vi "Split Registers by Direction.vi"(8 "error in":errorcluster, 11 "vi info":T1 {"RegisterMap"."Address" format="%.0x"}) -> (0 "error out":errorcluster, 2 "Controls":T8[](array[typedef]) {"Data Type" format="%.0x"}, 3 "Indicator":T8[](array[typedef]) {"Data Type" format="%.0x"})   [LabVIEW 2019, in "FPGA Addon System Explorer.lvlib"]
uses:
  FPGA Addon System Explorer.lvlib
  Shared/Register Information.ctl
  Shared/Data Type.ctl
  <vilib>/rvi/Bitfile/niFpgaBitfileStructure_VI.ctl
  <vilib>/rvi/Bitfile/nirviControlStructure.ctl
  <vilib>/rvi/Bitfile/nirviTypdefDescription.ctl
  <vilib>/rvi/Bitfile/nirviMechanicalAction.ctl
  <vilib>/rvi/Bitfile/nirviSubControlStructure.ctl
  <vilib>/rvi/Bitfile/nirviClusterElementControl.ctl
  <vilib>/picture/picture.llb/imagedata.ctl
  SubModules/FPGA Addon Speciality IO/Source/Types/PWM.Measure.Analog.Measurement.ctl
  SubModules/FPGA Addon Speciality IO/Source/Types/PWM.Measure.Digital.Measurement.ctl
  SubModules/FPGA Addon Speciality IO/Source/Types/Static.Measure.Digital.Measurement.ctl
  SubModules/FPGA Addon Speciality IO/Source/Types/QuadratureEncoder.Measure.Digital.Measurement.ctl
  SubModules/FPGA Addon Speciality IO/Source/Types/PWM.Generate.Digital.Settings.ctl
  SubModules/FPGA Addon Speciality IO/Source/Types/PWM.Measure.Analog.Settings.ctl
  SubModules/FPGA Addon Speciality IO/Source/Types/PWM.Measure.Digital.Settings.ctl
  SubModules/FPGA Addon Speciality IO/Source/Types/Sine.Generate.Settings.ctl
  SubModules/FPGA Addon Speciality IO/Source/Types/Static.Generate.Digital.Settings.ctl
  SubModules/FPGA Addon Speciality IO/Source/Types/Static.Measure.Digital.Settings.ctl
  SubModules/FPGA Addon Speciality IO/Source/Types/WSS.Generate.Digital.Settings.ctl
  SubModules/FPGA Addon Speciality IO/Source/Types/QuadratureEncoder.Measure.Digital.Settings.ctl
  Shared/FPGA Addon Shared.lvlib
  SubModules/FPGA Addon Speciality IO/Source/Speciality FPGA IO.lvlib
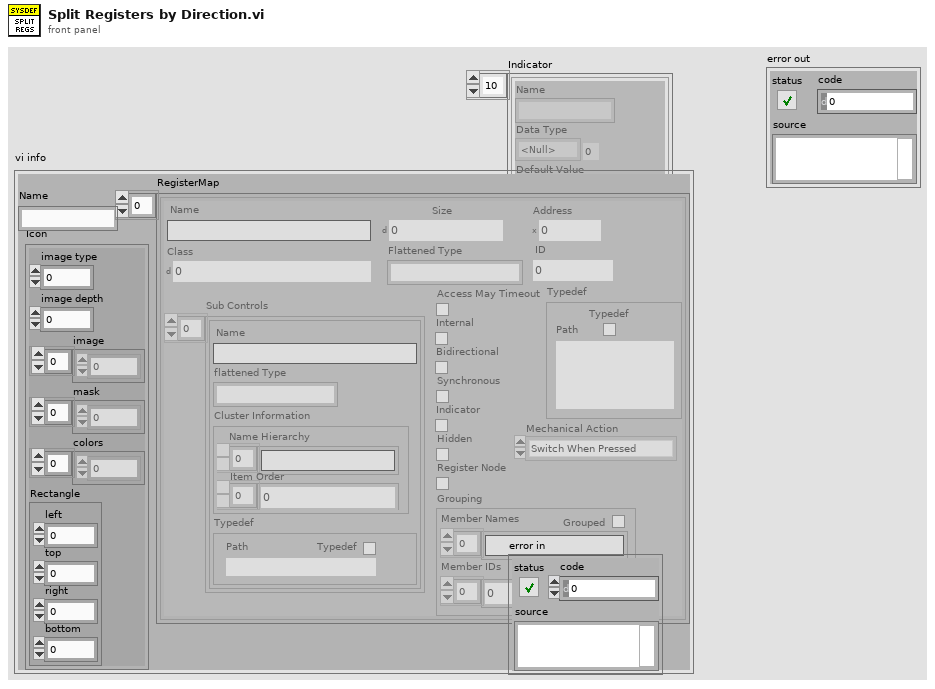
[diagram p1: front panel]
types:
  T1 = typedef "niFpgaBitfileStructure_VI.ctl" = cluster{"Name":string, "RegisterMap":T2[], "Icon":T7}
  T2 = typedef "nirviControlStructure.ctl" = cluster{"Name":string, "Hidden":bool, "Indicator":bool, "Flattened Type":string, "Grouping":cluster{"Grouped":bool, "Member Names":string[], "Member IDs":u32[]}, "Address":u32, "Size":u32, "Class":u32, "Internal":bool, "Typedef":T3, "ID":u32, "Bidirectional":bool, "Synchronous":bool, "Mechanical Action":T4, "Sub Controls":T5[], "Access May Timeout":bool, "Register Node":bool}
  T3 = typedef "nirviTypdefDescription.ctl" = cluster{"Typedef":bool, "Path":path}
  T4 = typedef "nirviMechanicalAction.ctl" = enum8{"Switch When Pressed", "Switch When Released", "Switch Until Released", "Latch When Pressed", "Latch When Released", "Latch Until Released"}
  T5 = typedef "nirviSubControlStructure.ctl" = cluster{"Name":string, "flattened Type":string, "Cluster Information":T6, "Typedef":T3}
  T6 = typedef "nirviClusterElementControl.ctl" = cluster{"Name Hierarchy":string[], "Item Order":u32[]}
  T7 = typedef "imagedata.ctl" = cluster{"image type":i32, "image depth":i32, "image":u8[], "mask":u8[], "colors":u32[], "Rectangle":cluster{"left":i16, "top":i16, "right":i16, "bottom":i16}}
  T8 = typedef "FPGA Addon Shared.lvlib/Register Information.ctl" = cluster{"Name":string, "Data Type":T9, "Default Value":variant}
  T9 = typedef "FPGA Addon Shared.lvlib/Data Type.ctl" = enum8{"<Null>", "I8", "I16", "I32", "I64", "U8", "U16", "U32", "U64", "SGL", "Boolean", "Analog PWM In Settings", "Analog PWM In", "Digital PWM In Settings", "Digital PWM In", "Digital PWM Out", "Sine Out", "FXP+/-24.5", "FXP+/-16.5", "FXP+/-32.8", "FXP+/-64.32", "FXP+/-16.7", "FXP+/-20.5", "FXP+/-27.5", "FXP+/-32.16", "FXP +16.3", "FXP +18.3", "Digital Static In", "Digital Static Out", "Digital Static In Settings", "Digital WSS Out", "Quad Encoder Settings", "Quad Encoder In"}
  T10 = typedef "Speciality FPGA IO.lvlib/QuadratureEncoder.Measure.Digital.Measurement.ctl" = cluster{"POSITION":i32}
  T11 = typedef "Speciality FPGA IO.lvlib/Static.Measure.Digital.Measurement.ctl" = cluster{"STATE":bool}
  T12 = typedef "Speciality FPGA IO.lvlib/PWM.Measure.Digital.Measurement.ctl" = cluster{"ACTIVE TICKS":u32, "INACTIVE TICKS":u32, "ACQ TICKS":u32}
  T13 = typedef "Speciality FPGA IO.lvlib/PWM.Measure.Analog.Measurement.ctl" = cluster{"ACTIVE TICKS":u32, "INACTIVE TICKS":u32, "ACQ TICKS":u32, "ACTIVE VOLTAGE":fxp<+/-,32,8>, "INACTIVE VOLTAGE":fxp<+/-,32,8>}
  T14 = typedef "Speciality FPGA IO.lvlib/QuadratureEncoder.Measure.Digital.Settings.ctl" = cluster{"DIRECTION":u8, "RESET VALUE":i32, "A RESET STATE":bool, "B RESET STATE":bool, "Z RESET STATE":bool}
  T15 = typedef "Speciality FPGA IO.lvlib/WSS.Generate.Digital.Settings.ctl" = cluster{"ACTIVE EDGE":bool, "ACTIVE TICKS":u32, "INACTIVE TICKS":u32, "DATA":u8, "SENSOR TYPE":u8}
  T16 = typedef "Speciality FPGA IO.lvlib/Static.Measure.Digital.Settings.ctl" = cluster{"ACTIVE EDGE":bool}
  T17 = typedef "Speciality FPGA IO.lvlib/Static.Generate.Digital.Settings.ctl" = cluster{"ACTIVE EDGE":bool, "OUTPUT":bool}
  T18 = typedef "Speciality FPGA IO.lvlib/Sine.Generate.Settings.ctl" = cluster{"AMP":fxp<+/-,32,8>, "OFFSET":fxp<+/-,32,8>, "PERIODS/TICKS":fxp<+,32,0>}
  T19 = typedef "Speciality FPGA IO.lvlib/PWM.Measure.Digital.Settings.ctl" = cluster{"ACTIVE EDGE":bool, "TIMEOUT":u32}
  T20 = typedef "Speciality FPGA IO.lvlib/PWM.Measure.Analog.Settings.ctl" = cluster{"ACTIVE EDGE":bool, "TIMEOUT":u32, "THRESHOLD":fxp<+/-,32,8>}
  T21 = typedef "Speciality FPGA IO.lvlib/PWM.Generate.Digital.Settings.ctl" = cluster{"ACTIVE EDGE":bool, "ACTIVE TICKS":u32, "INACTIVE TICKS":u32}
  T22 = typedef "Type Descriptor Enumeration__ogtk.ctl" = enum8{"<Null>", "I8", "I16", "I32", "I64", "U8", "U16", "U32", "U64", "SGL", "DBL", "EXT", "CSG", "CDB", "CXT", "0x0F", "0x10", "0x11", "0x12", "0x13", "0x14", "Enum U8", "Enum U16", "Enum U32", "Enum U64", "SGL PQ", "DBL PQ", "EXT PQ", "CSG PQ", "CDB PQ", "CXT PQ", "0x1F", "0x20", "Boolean", "0x22", "0x23", "0x24", "0x25", "0x26", "0x27", "0x28", "0x29", "0x2A", "0x2B", "0x2C", "0x2D", "0x2E", "0x2F", "String", "0x31", "Path", "Pict", "0x34", "0x35", "0x36", "DAQ", "0x38", "0x39", "0x3A", "0x3B", "0x3C", "0x3D", "0x3E", "0x3F", "Array", "0x41", "0x42", "0x43", "0x44", "0x45", "0x46", "0x47", "0x48", "0x49", "0x4A", "0x4B", "0x4C", "0x4D", "0x4E", "0x4F", "Cluster", "0x51", "0x52", "Variant", "Waveform", "0x55", "0x56", "0x57", "0x58", "0x59", "0x5A", "0x5B", "0x5C", "0x5D", "0x5E", "0x5F", "0x60", "0x61", "0x62", "0x63", "0x64", "0x65", "0x66", "0x67", "0x68", "0x69", "0x6A", "0x6B", "0x6C", "0x6D", "0x6E", "0x6F", "Refnum"}
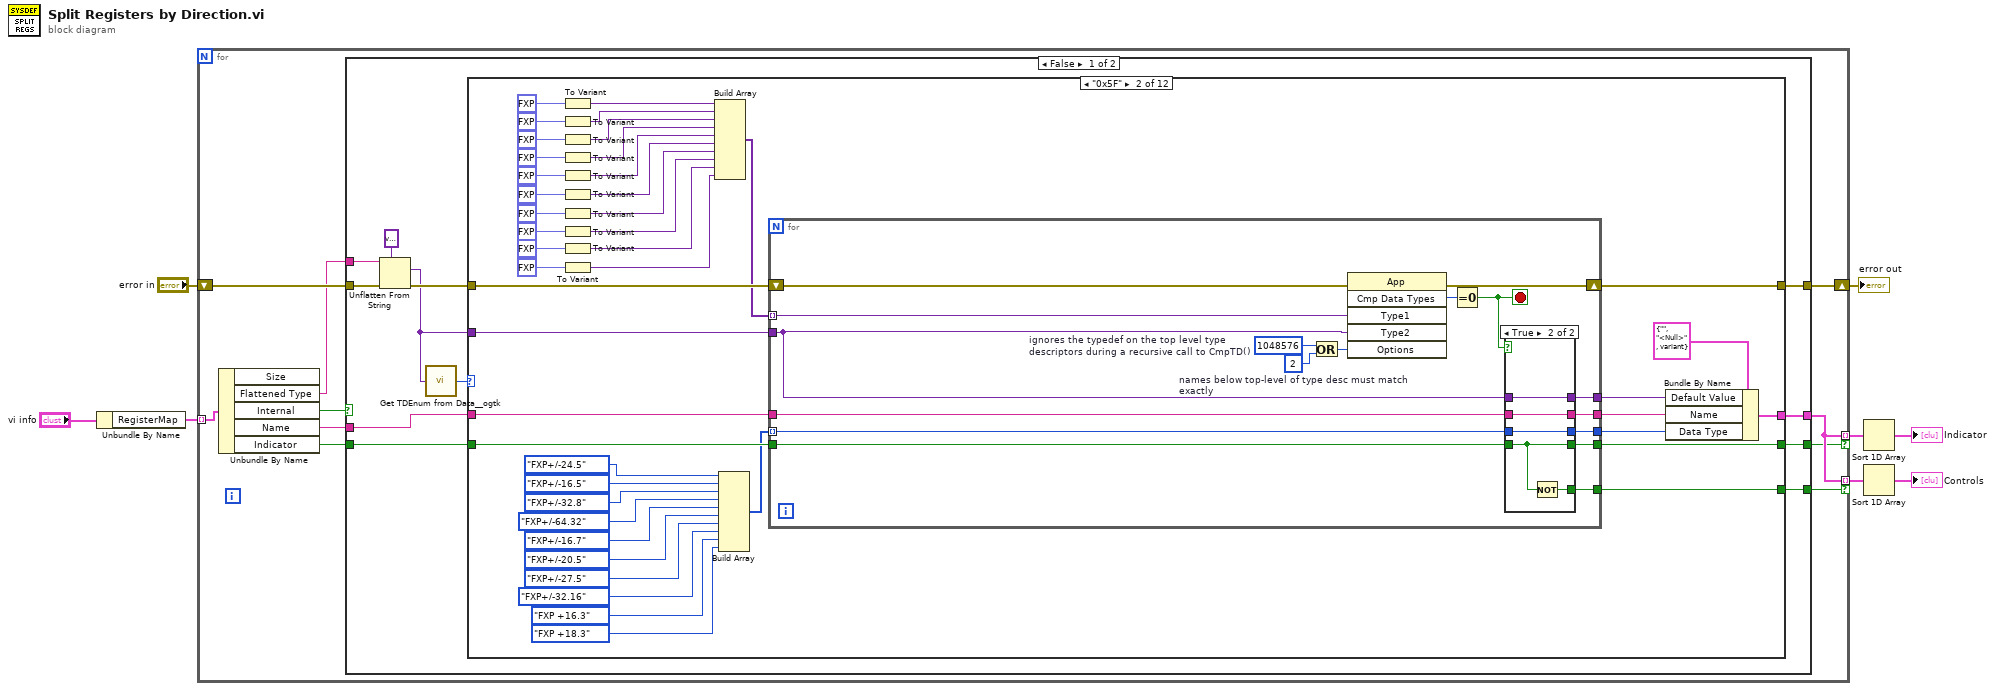
[diagram p0: block diagram]
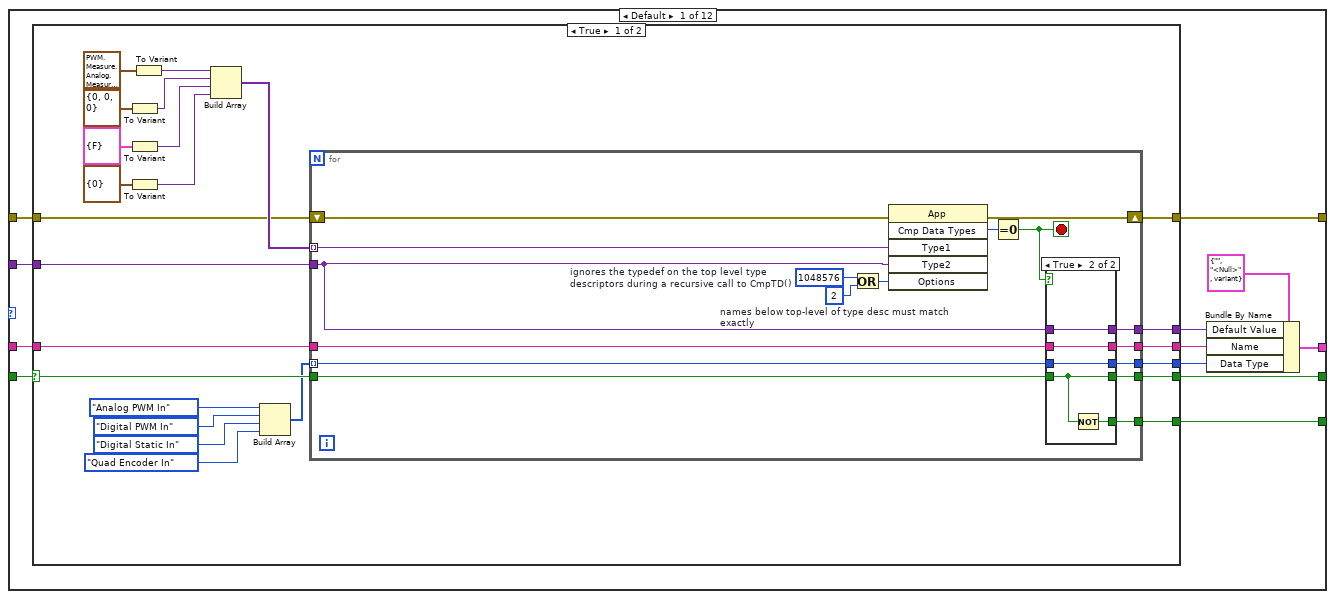
[diagram p2: hidden frame]
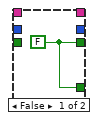
[diagram p3: hidden frame]
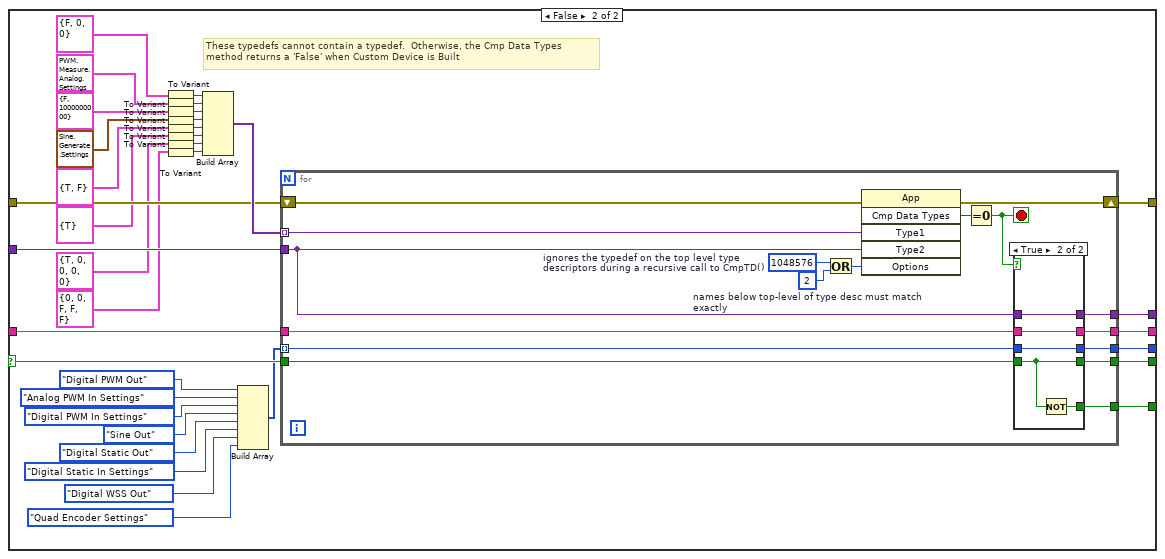
[diagram p4: hidden frame]
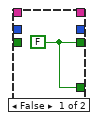
[diagram p5: hidden frame]
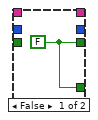
[diagram p6: hidden frame]
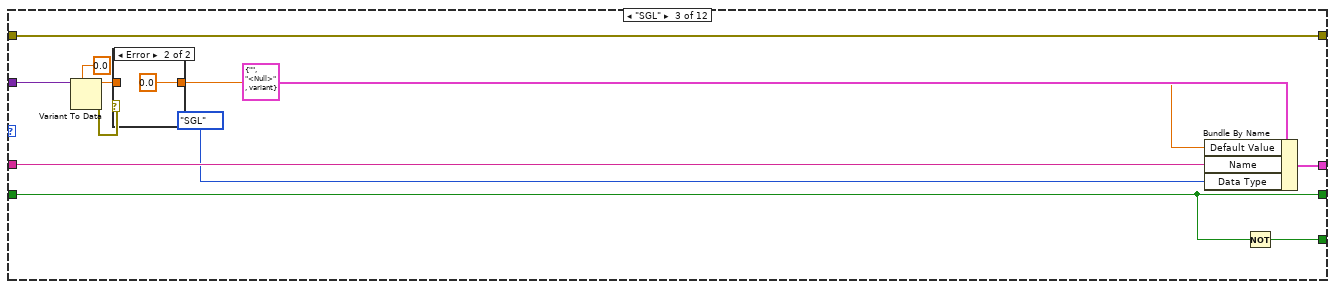
[diagram p7: hidden frame]
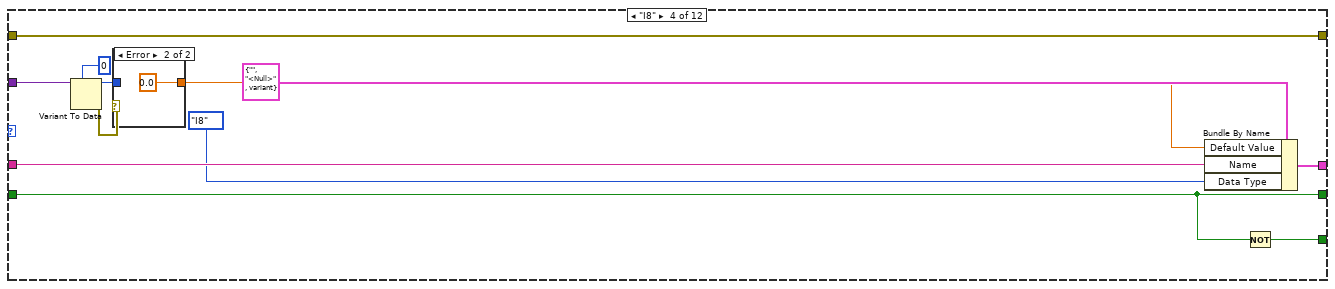
[diagram p9: hidden frame]
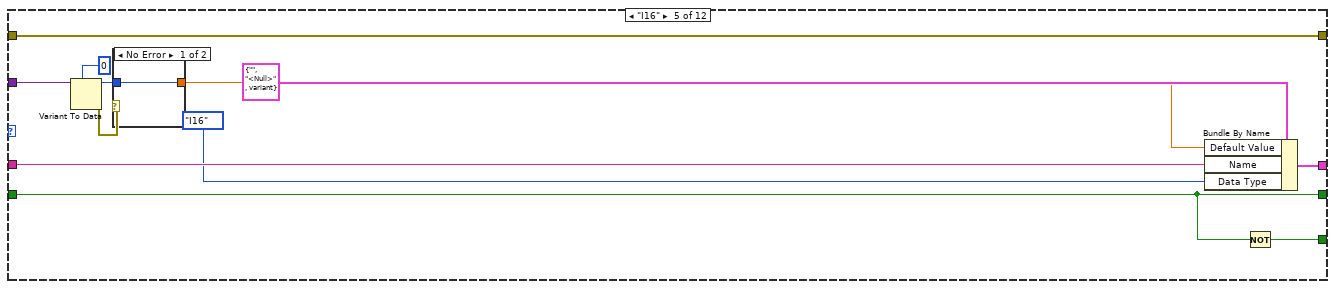
[diagram p11: hidden frame]
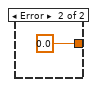
[diagram p12: hidden frame]
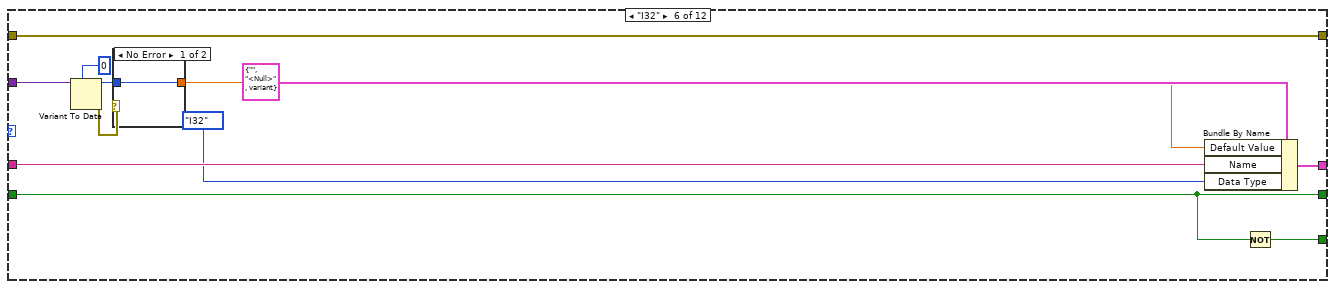
[diagram p13: hidden frame]
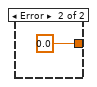
[diagram p14: hidden frame]
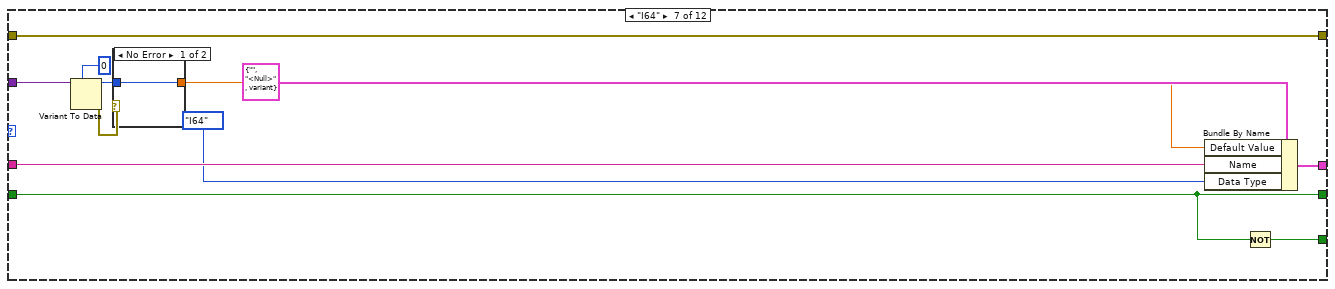
[diagram p15: hidden frame]
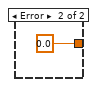
[diagram p16: hidden frame]
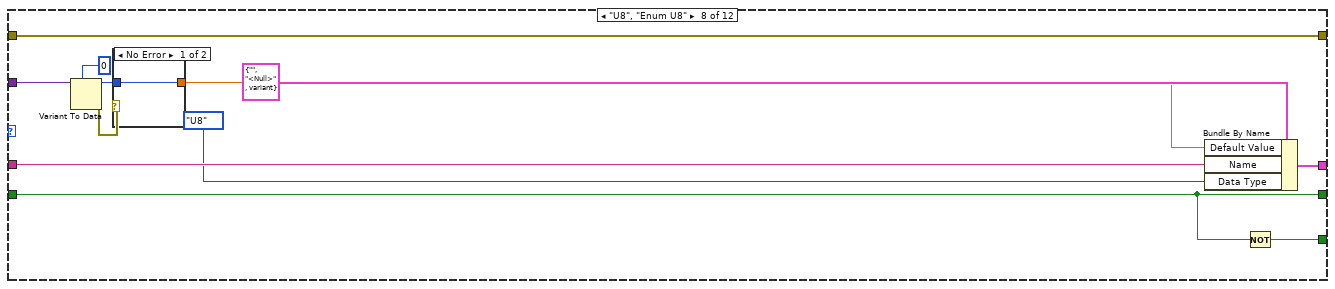
[diagram p17: hidden frame]
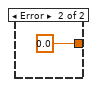
[diagram p18: hidden frame]
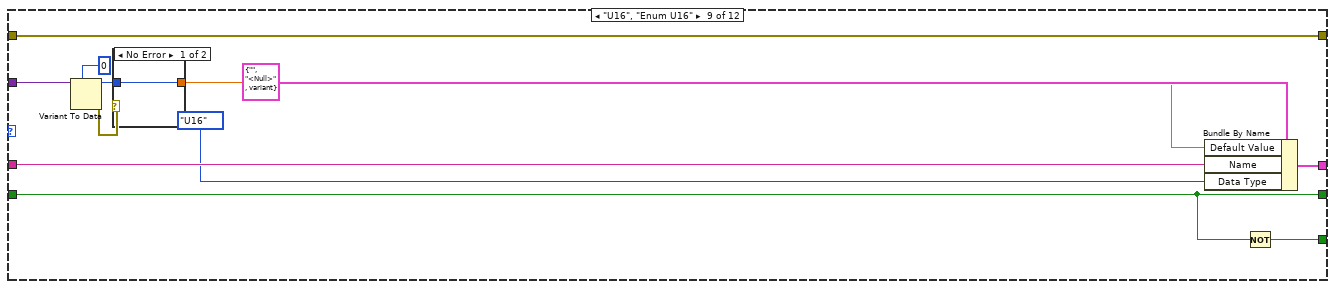
[diagram p19: hidden frame]
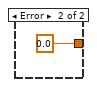
[diagram p20: hidden frame]
diagram:
  n1 = Unbundle By Name("vi info") -> ("RegisterMap"=w6:T2[])
  n2 = for {
    tunnel: w6 -> [w13] mode=indexing
    tunnel: [w18] -> w7 mode=indexing if=w17
    tunnel: [w18] -> w8 mode=indexing if=w16
    shift-right: [w15] -> w2
    shift-left: "error in" -> [w14]
    n3 = Unbundle By Name(w13) -> ("Flattened Type"=w9:string, "Internal"=w10:bool, "Name"=w11:string, "Indicator"=w12:bool)  [unwired: 1 out]
    n4 = case shown="False" w10 {
      tunnel: w11 -> [w29 _]
      tunnel: w12 -> [w28 _]
      tunnel: [w27 _] -> w18
      tunnel: [w26 w358] -> w17
      tunnel: [w25 w358] -> w16
      tunnel: w9 -> [w22 _]
      tunnel: [w24 w357] -> w15
      tunnel: w14 -> [w21 w357]
      frame False {
        n5 = Unflatten From String(type=variant ("Variant"), binary string=w22, error in (no error)=w21) -> (value=w19:variant, error out=w20:errorcluster)  [unwired: 3 out]
        n6 = call <userlib>:"Get TDEnum from Data__ogtk.vi"("Data"=w19) -> ("Type Descriptor Enumeration"=w30:T22)  [unwired: 4 in]
        n7 = case shown="\"0x5F\"" w30 {
          tunnel: [w42 w192 w224 w238 w252 w266 w280 w294 w308 w322 w336 w350] -> w26
          tunnel: w28 -> [w37 w187 w224 w238 w252 w266 w280 w294 w308 w322 w336 w350]
          tunnel: w29 -> [w38 w188 w226 w240 w254 w268 w282 w296 w310 w324 w338 w352]
          tunnel: [w39 w189 w225 w239 w253 w267 w281 w295 w309 w323 w337 w351] -> w27
          tunnel: [w41 w191 w223 w237 w251 w265 w279 w293 w307 w321 w335 w349] -> w25
          tunnel: w19 -> [w36 w186 w222 w236 w250 w264 w278 w292 w306 w320 w334 w348]
          tunnel: [w32 w182 w216 w230 w244 w258 w272 w286 w300 w314 w328 w342] -> w24
          tunnel: w20 -> [w31 w181 w216 w230 w244 w258 w272 w286 w300 w314 w328 w342]
          frame Default {
            n8 = case shown="True" w37 {
              selector: w37 -> [w61 w121]
              tunnel: [w66 w125] -> w42
              tunnel: [w65 w124] -> w41
              tunnel: w38 -> [w64 w123]
              tunnel: w36 -> [w55 w117]
              tunnel: [w54 w116] -> w35
              tunnel: [w53 w115] -> w34
              tunnel: [w52 w114] -> w33
              tunnel: [w50 w105] -> w32
              tunnel: w31 -> [w49 w106]
              frame True {
                n9 = To Variant(anything=T12 {"ACTIVE TICKS"=0, "INACTIVE TICKS"=0, "ACQ TICKS"=0} ("Cached.Data")) -> (Variant=w59:variant)
                n10 = To Variant(anything=T11 {"STATE"=FALSE} ("Cached.Data")) -> (Variant=w47:variant)
                n11 = To Variant(anything=T10 {"POSITION"=0} ("Cached.Data")) -> (Variant=w43:variant)
                n12 = To Variant(anything=T13 {"ACTIVE TICKS"=0, "INACTIVE TICKS"=0, "ACQ TICKS"=0, "ACTIVE VOLTAGE"=0.0, "INACTIVE VOLTAGE"=0.0} ("Cached.Data")) -> (Variant=w60:variant)
                n13 = Build Array(w60, w59, w47, w43) -> (w56:variant[])
                n14 = Build Array(Data_Type."Analog PWM In" ("Data Type"), Data_Type."Digital PWM In" ("Data Type"), Data_Type."Digital Static In" ("Data Type"), Data_Type."Quad Encoder In" ("Data Type")) -> (w51:T9[])
                n15 = for {
                  tunnel: w55 -> [w70]
                  tunnel: [w81] -> w65
                  tunnel: w64 -> [w80]
                  tunnel: w56 -> [w72] mode=indexing
                  tunnel: [w79] -> w53
                  tunnel: [w78] -> w54
                  tunnel: [w77] -> w52
                  tunnel: w51 -> [w76] mode=indexing
                  tunnel: w61 -> [w83]
                  tunnel: [w82] -> w66
                  shift-right: [w67] -> w50
                  shift-left: w49 -> [w68]
                  stop <- w71 stop-if-true
                  w69 = 2  # names below top-level of type desc must match exactly
                  w74 = 1048576  # ignores the typedef on the top level type descriptors during a recursive call to CmpTD()
                  n16 = Or(x=w74, y=w69) -> (x .or. y?=w75:i32)
                  n17 = invoke class="App" method="Cmp Data Types"(error in=w68, "Type1"=w72, "Type2"=w70, "Options"=w75) -> (error out=w67:errorcluster, "Compare Data Types"=w73:i32)  [unwired: 2 in, 4 out]
                  n18 = Equal To 0?(x=w73) -> (x = 0?=w71:bool)
                  n19 = case shown="True" w71 {
                    tunnel: w83 -> [_ w89]
                    tunnel: [w84 w89] -> w82
                    tunnel: [w84 w88] -> w81
                    tunnel: w80 -> [_ w86]
                    tunnel: [_ w87] -> w79
                    tunnel: w70 -> [_ w87]
                    tunnel: [_ w86] -> w78
                    tunnel: [_ w85] -> w77
                    tunnel: w76 -> [_ w85]
                    frame False {
                      w84 = FALSE ("Boolean")
                    }
                    frame True {
                      n20 = Not(x=w89) -> (.not. x?=w88:bool)
                    }
                  }
                }
              }
              frame False {
                # "These typedefs cannot contain a typedef.  Otherwise, the Cmp Data Types \nmethod returns a 'False' when Custom Device is Built"
                n21 = To Variant(anything=T21 {"ACTIVE EDGE"=FALSE, "ACTIVE TICKS"=0, "INACTIVE TICKS"=0} ("Channel.Settings")) -> (Variant=w120:variant)
                n22 = To Variant(anything=T20 {"ACTIVE EDGE"=FALSE, "TIMEOUT"=1000000000, "THRESHOLD"=3.0} ("Channel.Settings")) -> (Variant=w110:variant)
                n23 = To Variant(anything=T19 {"ACTIVE EDGE"=FALSE, "TIMEOUT"=1000000000} ("Channel.Settings")) -> (Variant=w109:variant)
                n24 = To Variant(anything=T18 {"AMP"=0.0, "OFFSET"=0.0, "PERIODS/TICKS"=0.0002500000409781933} ("Settings")) -> (Variant=w103:variant)
                n25 = To Variant(anything=T17 {"ACTIVE EDGE"=TRUE, "OUTPUT"=FALSE} ("Settings")) -> (Variant=w101:variant)
                n26 = To Variant(anything=T16 {"ACTIVE EDGE"=TRUE} ("Settings")) -> (Variant=w98:variant)
                n27 = To Variant(anything=T15 {"ACTIVE EDGE"=TRUE, "ACTIVE TICKS"=0, "INACTIVE TICKS"=0, "DATA"=0, "SENSOR TYPE"=0} ("Wheel Speed Sensor Settings")) -> (Variant=w94:variant)
                n28 = To Variant(anything=T14 {"DIRECTION"=0, "RESET VALUE"=0, "A RESET STATE"=FALSE, "B RESET STATE"=FALSE, "Z RESET STATE"=FALSE} ("Settings")) -> (Variant=w91:variant)
                n29 = Build Array(w120, w110, w109, w103, w101, w98, w94, w91) -> (w118:variant[])
                n30 = Build Array(Data_Type."Digital PWM Out" ("Data Type"), Data_Type."Analog PWM In Settings" ("Data Type"), Data_Type."Digital PWM In Settings" ("Data Type"), Data_Type."Sine Out" ("Data Type"), Data_Type."Digital Static Out" ("Data Type"), Data_Type."Digital Static In Settings" ("Data Type"), Data_Type."Digital WSS Out" ("Data Type"), Data_Type."Quad Encoder Settings" ("Data Type")) -> (w113:T9[])
                n31 = for {
                  tunnel: w117 -> [w131]
                  tunnel: [w140] -> w124
                  tunnel: w123 -> [w139]
                  tunnel: w118 -> [w130] mode=indexing
                  tunnel: [w138] -> w115
                  tunnel: [w137] -> w116
                  tunnel: [w136] -> w114
                  tunnel: w113 -> [w135] mode=indexing
                  tunnel: w121 -> [w142]
                  tunnel: [w141] -> w125
                  shift-right: [w126] -> w105
                  shift-left: w106 -> [w127]
                  stop <- w128 stop-if-true
                  w133 = 2  # names below top-level of type desc must match exactly
                  w132 = 1048576  # ignores the typedef on the top level type descriptors during a recursive call to CmpTD()
                  n32 = Or(x=w132, y=w133) -> (x .or. y?=w134:i32)
                  n33 = invoke class="App" method="Cmp Data Types"(error in=w127, "Type1"=w130, "Type2"=w131, "Options"=w134) -> (error out=w126:errorcluster, "Compare Data Types"=w129:i32)  [unwired: 2 in, 4 out]
                  n34 = Equal To 0?(x=w129) -> (x = 0?=w128:bool)
                  n35 = case shown="True" w128 {
                    tunnel: w142 -> [_ w148]
                    tunnel: [w143 w148] -> w141
                    tunnel: [w143 w147] -> w140
                    tunnel: w139 -> [_ w145]
                    tunnel: [_ w146] -> w138
                    tunnel: w131 -> [_ w146]
                    tunnel: [_ w145] -> w137
                    tunnel: [_ w144] -> w136
                    tunnel: w135 -> [_ w144]
                    frame False {
                      w143 = FALSE ("Boolean")
                    }
                    frame True {
                      n36 = Not(x=w148) -> (.not. x?=w147:bool)
                    }
                  }
                }
              }
            }
            n37 = Bundle By Name(cluster=T8 {"Name"="", "Data Type"=enum."<Null>", "Default Value"=variant(refnum<class> refnum)}, "Default Value"=w34, "Name"=w35, "Data Type"=w33) -> (w39:T8)
          }
          frame "0x5F" {
            n38 = To Variant(anything=fxp<+/-,24,5> 0.0 ("Numeric 1 In")) -> (Variant=w180:variant)
            n39 = To Variant(anything=fxp<+/-,16,5> 0.0 ("Numeric 2 In")) -> (Variant=w179:variant)
            n40 = To Variant(anything=fxp<+/-,32,8> 0.0 ("Numeric 3 In")) -> (Variant=w172:variant)
            n41 = To Variant(anything=fxp<+/-,64,32> 0.0 ("Numeric 4 In")) -> (Variant=w171:variant)
            n42 = To Variant(anything=fxp<+/-,16,7> 0.0 ("Numeric 4 In")) -> (Variant=w165:variant)
            n43 = To Variant(anything=fxp<+/-,20,5> 0.0 ("Numeric 4 In")) -> (Variant=w162:variant)
            n44 = To Variant(anything=fxp<+/-,27,5> 0.0 ("Numeric 4 In")) -> (Variant=w159:variant)
            n45 = To Variant(anything=fxp<+/-,32,16> 0.0 ("Numeric 4 In")) -> (Variant=w156:variant)
            n46 = To Variant(anything=fxp<+,16,3> 0.0 ("Numeric 4 In")) -> (Variant=w153:variant)
            n47 = To Variant(anything=fxp<+,18,3> 0.0 ("Numeric 4 In")) -> (Variant=w151:variant)
            n48 = Build Array(w180, w179, w172, w171, w165, w162, w159, w156, w153, w151) -> (w176:variant[])
            n49 = Build Array(Data_Type."FXP+/-24.5" ("Data Type"), Data_Type."FXP+/-16.5" ("Data Type"), Data_Type."FXP+/-32.8" ("Data Type"), Data_Type."FXP+/-64.32" ("Data Type"), Data_Type."FXP+/-16.7" ("Data Type"), Data_Type."FXP+/-20.5" ("Data Type"), Data_Type."FXP+/-27.5" ("Data Type"), Data_Type."FXP+/-32.16" ("Data Type"), Data_Type."FXP +16.3" ("Data Type"), Data_Type."FXP +18.3" ("Data Type")) -> (w175:T9[])
            n50 = for {
              tunnel: w186 -> [w196]
              tunnel: [w207] -> w191
              tunnel: w188 -> [w206]
              tunnel: w176 -> [w198] mode=indexing
              tunnel: [w205] -> w184
              tunnel: [w204] -> w185
              tunnel: [w203] -> w183
              tunnel: w175 -> [w202] mode=indexing
              tunnel: w187 -> [w209]
              tunnel: [w208] -> w192
              shift-right: [w193] -> w182
              shift-left: w181 -> [w194]
              stop <- w197 stop-if-true
              w195 = 2  # names below top-level of type desc must match exactly
              w200 = 1048576  # ignores the typedef on the top level type descriptors during a recursive call to CmpTD()
              n51 = Or(x=w200, y=w195) -> (x .or. y?=w201:i32)
              n52 = invoke class="App" method="Cmp Data Types"(error in=w194, "Type1"=w198, "Type2"=w196, "Options"=w201) -> (error out=w193:errorcluster, "Compare Data Types"=w199:i32)  [unwired: 2 in, 4 out]
              n53 = Equal To 0?(x=w199) -> (x = 0?=w197:bool)
              n54 = case shown="True" w197 {
                tunnel: w209 -> [_ w215]
                tunnel: [w210 w215] -> w208
                tunnel: [w210 w214] -> w207
                tunnel: w206 -> [_ w212]
                tunnel: [_ w213] -> w205
                tunnel: w196 -> [_ w213]
                tunnel: [_ w212] -> w204
                tunnel: [_ w211] -> w203
                tunnel: w202 -> [_ w211]
                frame False {
                  w210 = FALSE ("Boolean")
                }
                frame True {
                  n55 = Not(x=w215) -> (.not. x?=w214:bool)
                }
              }
            }
            n56 = Bundle By Name(cluster=T8 {"Name"="", "Data Type"=enum."<Null>", "Default Value"=variant(refnum<class> refnum)}, "Default Value"=w184, "Name"=w185, "Data Type"=w183) -> (w189:T8)
          }
          frame "SGL" {
            n57 = Variant To Data(type=sgl 0.0, Variant=w222) -> (data=w218:sgl, error out=w220:errorcluster)  [unwired: 1 in]
            n58 = case shown="Error" w220 {
              tunnel: [w228 0.0] -> w219
              tunnel: w218 -> [w228 _]
              frame No Error {
              }
              frame Error {
              }
            }
            n59 = Bundle By Name(cluster=T8 {"Name"="", "Data Type"=enum."<Null>", "Default Value"=variant(refnum<class> refnum)}, "Default Value"=w219, "Name"=w226, "Data Type"=Data_Type."SGL") -> (w225:T8)
            n60 = Not(x=w224) -> (.not. x?=w223:bool)
          }
          frame "I8" {
            n61 = Variant To Data(type=i8 0, Variant=w236) -> (data=w232:i8, error out=w234:errorcluster)  [unwired: 1 in]
            n62 = case shown="Error" w234 {
              tunnel: [w242 0.0] -> w233
              tunnel: w232 -> [w242 _]
              frame No Error {
              }
              frame Error {
              }
            }
            n63 = Bundle By Name(cluster=T8 {"Name"="", "Data Type"=enum."<Null>", "Default Value"=variant(refnum<class> refnum)}, "Default Value"=w233, "Name"=w240, "Data Type"=Data_Type."I8") -> (w239:T8)
            n64 = Not(x=w238) -> (.not. x?=w237:bool)
          }
          frame "I16" {
            n65 = Variant To Data(type=i16 0, Variant=w250) -> (data=w246:i16, error out=w248:errorcluster)  [unwired: 1 in]
            n66 = case shown="No Error" w248 {
              tunnel: [w256 0.0] -> w247
              tunnel: w246 -> [w256 _]
              frame No Error {
              }
              frame Error {
              }
            }
            n67 = Bundle By Name(cluster=T8 {"Name"="", "Data Type"=enum."<Null>", "Default Value"=variant(refnum<class> refnum)}, "Default Value"=w247, "Name"=w254, "Data Type"=Data_Type."I16") -> (w253:T8)
            n68 = Not(x=w252) -> (.not. x?=w251:bool)
          }
          frame "I32" {
            n69 = Variant To Data(type=0, Variant=w264) -> (data=w260:i32, error out=w262:errorcluster)  [unwired: 1 in]
            n70 = case shown="No Error" w262 {
              tunnel: [w270 0.0] -> w261
              tunnel: w260 -> [w270 _]
              frame No Error {
              }
              frame Error {
              }
            }
            n71 = Bundle By Name(cluster=T8 {"Name"="", "Data Type"=enum."<Null>", "Default Value"=variant(refnum<class> refnum)}, "Default Value"=w261, "Name"=w268, "Data Type"=Data_Type."I32") -> (w267:T8)
            n72 = Not(x=w266) -> (.not. x?=w265:bool)
          }
          frame "I64" {
            n73 = Variant To Data(type=i64 0, Variant=w278) -> (data=w274:i64, error out=w276:errorcluster)  [unwired: 1 in]
            n74 = case shown="No Error" w276 {
              tunnel: [w284 0.0] -> w275
              tunnel: w274 -> [w284 _]
              frame No Error {
              }
              frame Error {
              }
            }
            n75 = Bundle By Name(cluster=T8 {"Name"="", "Data Type"=enum."<Null>", "Default Value"=variant(refnum<class> refnum)}, "Default Value"=w275, "Name"=w282, "Data Type"=Data_Type."I64") -> (w281:T8)
            n76 = Not(x=w280) -> (.not. x?=w279:bool)
          }
          frame "U8", "Enum U8" {
            n77 = Variant To Data(type=u8 0, Variant=w292) -> (data=w288:u8, error out=w290:errorcluster)  [unwired: 1 in]
            n78 = case shown="No Error" w290 {
              tunnel: [w298 0.0] -> w289
              tunnel: w288 -> [w298 _]
              frame No Error {
              }
              frame Error {
              }
            }
            n79 = Bundle By Name(cluster=T8 {"Name"="", "Data Type"=enum."<Null>", "Default Value"=variant(refnum<class> refnum)}, "Default Value"=w289, "Name"=w296, "Data Type"=Data_Type."U8") -> (w295:T8)
            n80 = Not(x=w294) -> (.not. x?=w293:bool)
          }
          frame "U16", "Enum U16" {
            n81 = Variant To Data(type=u16 0, Variant=w306) -> (data=w302:u16, error out=w304:errorcluster)  [unwired: 1 in]
            n82 = case shown="No Error" w304 {
              tunnel: [w312 0.0] -> w303
              tunnel: w302 -> [w312 _]
              frame No Error {
              }
              frame Error {
              }
            }
            n83 = Bundle By Name(cluster=T8 {"Name"="", "Data Type"=enum."<Null>", "Default Value"=variant(refnum<class> refnum)}, "Default Value"=w303, "Name"=w310, "Data Type"=Data_Type."U16") -> (w309:T8)
            n84 = Not(x=w308) -> (.not. x?=w307:bool)
          }
          frame "U32", "Enum U32" {
            n85 = Variant To Data(type=u32 0, Variant=w320) -> (data=w316:u32, error out=w318:errorcluster)  [unwired: 1 in]
            n86 = case shown="No Error" w318 {
              tunnel: [w326 0.0] -> w317
              tunnel: w316 -> [w326 _]
              frame No Error {
              }
              frame Error {
              }
            }
            n87 = Bundle By Name(cluster=T8 {"Name"="", "Data Type"=enum."<Null>", "Default Value"=variant(refnum<class> refnum)}, "Default Value"=w317, "Name"=w324, "Data Type"=Data_Type."U32") -> (w323:T8)
            n88 = Not(x=w322) -> (.not. x?=w321:bool)
          }
          frame "U64", "Enum U64" {
            n89 = Variant To Data(type=u64 0, Variant=w334) -> (data=w330:u64, error out=w332:errorcluster)  [unwired: 1 in]
            n90 = case shown="No Error" w332 {
              tunnel: [w340 0.0] -> w331
              tunnel: w330 -> [w340 _]
              frame No Error {
              }
              frame Error {
              }
            }
            n91 = Bundle By Name(cluster=T8 {"Name"="", "Data Type"=enum."<Null>", "Default Value"=variant(refnum<class> refnum)}, "Default Value"=w331, "Name"=w338, "Data Type"=Data_Type."U64") -> (w337:T8)
            n92 = Not(x=w336) -> (.not. x?=w335:bool)
          }
          frame "Boolean" {
            n93 = Variant To Data(type=FALSE, Variant=w348) -> (data=w344:bool, error out=w346:errorcluster)  [unwired: 1 in]
            n94 = case shown="No Error" w346 {
              tunnel: [w354 0.0] -> w345
              tunnel: w344 -> [w355 _]
              frame No Error {
                n95 = Boolean To (0,1)(Boolean=w355) -> (0, 1=w354:i16)
              }
              frame Error {
              }
            }
            n96 = Bundle By Name(cluster=T8 {"Name"="", "Data Type"=enum."<Null>", "Default Value"=variant(refnum<class> refnum)}, "Default Value"=w345, "Name"=w352, "Data Type"=Data_Type."Boolean") -> (w351:T8)
            n97 = Not(x=w350) -> (.not. x?=w349:bool)
          }
        }
      }
      frame True {
        w358 = FALSE ("Boolean")
      }
    }
  }
  "error out" <- w2
  n98 = Sort 1D Array(array=w7) -> (sorted array=→"Indicator":T8[])
  n99 = Sort 1D Array(array=w8) -> (sorted array=→"Controls":T8[])
